vi "hammerbot blue.vi"   [LabVIEW 2010, in "HammerBot.lvrbt"]
uses:
  HammerBot.lvrbt
  <vilib>/NXT/Subs/MotorOutput.ctl
  <vilib>/NXT/Block Support/NXT_MessageMailbox.ctl
  <vilib>/NXT/Dual Mode Library/Motors/ResetMotor.vi
  <vilib>/NXT/Dual Mode Library/Motors/MotorOn.vi
  <vilib>/NXT/Dual Mode Library/Motors/Rotation.vi
  <vilib>/NXT/Dual Mode Library/Motors/MotorBrake.vi
  <vilib>/NXT/Dual Mode Library/Motors/MotorReverse.vi
types:
  T1 = typedef "MotorOutput.ctl" = u8
  T2 = typedef "NXT_MessageMailbox.ctl" = u8
  T3 = typedef "LVHSConnector.ctl" = cluster{"Hardware":string, "Flattened String":string}
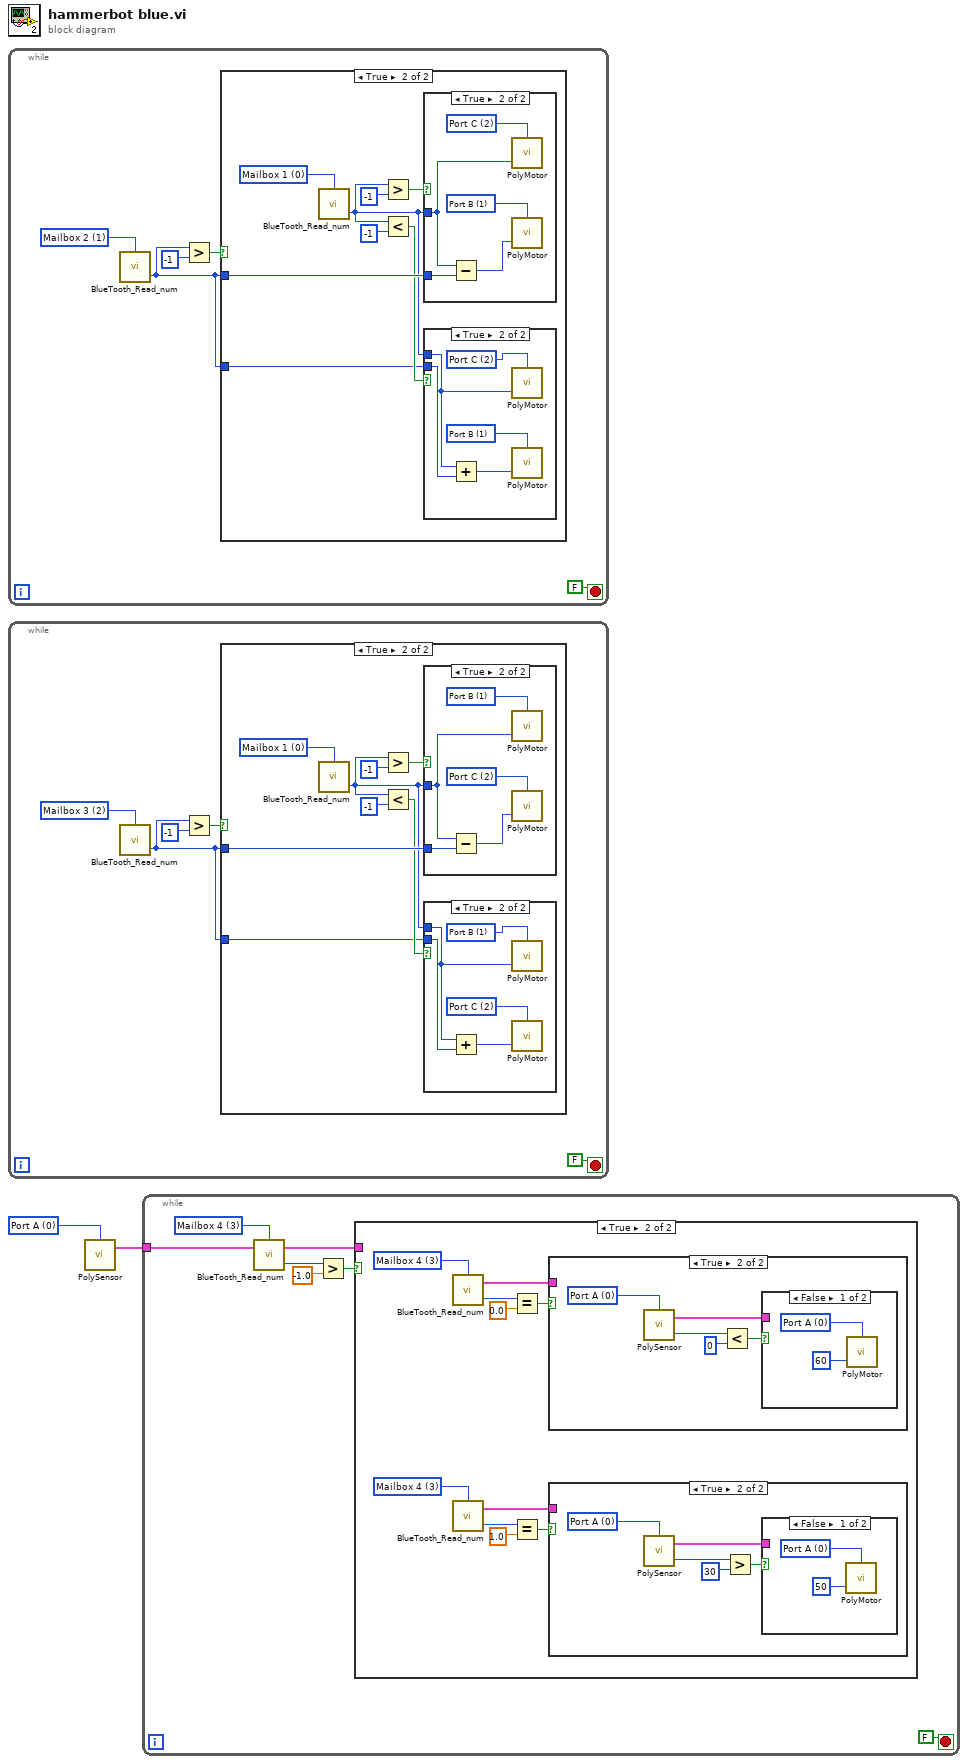
[diagram p0: block diagram]
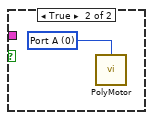
[diagram p10: hidden frame]
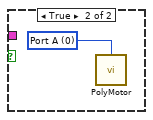
[diagram p12: hidden frame]
diagram:
  w1 = T1 0 items=["Port A"=0, "Port B"=1, "Port C"=2, "Ports A & B"=4, "Ports A & C"=5, "Ports B & C"=6, "All Ports"=3] ("Port (All Ports)")
  n1 = while {
    stop <- FALSE stop-if-true
    w7 = T2 1 items=["Mailbox 1", "Mailbox 2", "Mailbox 3", "Mailbox 4", "Mailbox 5", "Mailbox 6", "Mailbox 7", "Mailbox 8", "Mailbox 9", "Mailbox 10"] ("Mailbox")
    n2 = call <vilib>:"BlueTooth_Read_num.vi"("Mailbox"=w7) -> ("Message"=w3:i32)  [unwired: 2 in, 1 out]
    n3 = Greater?(x=w3, y=-1) -> (0:w5:bool)
    n4 = case shown="True" w5 {
      tunnel: w3 -> [_ w14]
      tunnel: w3 -> [_ w8]
      frame False {
      }
      frame True {
        w15 = T2 0 items=["Mailbox 1", "Mailbox 2", "Mailbox 3", "Mailbox 4", "Mailbox 5", "Mailbox 6", "Mailbox 7", "Mailbox 8", "Mailbox 9", "Mailbox 10"] ("Mailbox")
        n5 = call <vilib>:"BlueTooth_Read_num.vi"("Mailbox"=w15) -> ("Message"=w13:i32)  [unwired: 2 in, 1 out]
        n6 = Greater?(x=w13, y=-1) -> (0:w10:bool)
        n7 = Less?(x=w13, y=-1) -> (x < y?=w9:bool)
        n8 = case shown="True" w10 {
          tunnel: w13 -> [_ w24]
          tunnel: w14 -> [_ w21]
          frame False {
          }
          frame True {
            w25 = T1 1 items=["Port A"=0, "Port B"=1, "Port C"=2, "Ports A & B"=4, "Ports A & C"=5, "Ports B & C"=6, "All Ports"=3] ("Output Port (All Ports)")
            w22 = T1 2 items=["Port A"=0, "Port B"=1, "Port C"=2, "Ports A & B"=4, "Ports A & C"=5, "Ports B & C"=6, "All Ports"=3] ("Output Port (All Ports)")
            n9 = Subtract(x=w24, y=w21) -> (x-y=w23:i32)
            n10 = call-poly <vilib>:"PolyMotor.vi"("Power (75)"=w24, "Output Port (All Ports)"=w22) -> ()  [unwired: 2 in, 1 out]
            n11 = call-poly <vilib>:"PolyMotor.vi"("Power (75)"=w23, "Output Port (All Ports)"=w25) -> ()  [unwired: 2 in, 1 out]
          }
        }
        n12 = case shown="True" w9 {
          tunnel: w13 -> [_ w17]
          tunnel: w8 -> [_ w16]
          frame False {
          }
          frame True {
            w20 = T1 1 items=["Port A"=0, "Port B"=1, "Port C"=2, "Ports A & B"=4, "Ports A & C"=5, "Ports B & C"=6, "All Ports"=3] ("Output Port (All Ports)")
            w18 = T1 2 items=["Port A"=0, "Port B"=1, "Port C"=2, "Ports A & B"=4, "Ports A & C"=5, "Ports B & C"=6, "All Ports"=3] ("Output Port (All Ports)")
            n13 = Add(x=w17, y=w16) -> (x+y=w19:i32)
            n14 = call-poly <vilib>:"PolyMotor.vi"("Power (75)"=w17, "Output Port (All Ports)"=w18) -> ()  [unwired: 2 in, 1 out]
            n15 = call-poly <vilib>:"PolyMotor.vi"("Power (75)"=w19, "Output Port (All Ports)"=w20) -> ()  [unwired: 2 in, 1 out]
          }
        }
      }
    }
  }
  n16 = while {
    stop <- FALSE stop-if-true
    w30 = T2 2 items=["Mailbox 1", "Mailbox 2", "Mailbox 3", "Mailbox 4", "Mailbox 5", "Mailbox 6", "Mailbox 7", "Mailbox 8", "Mailbox 9", "Mailbox 10"] ("Mailbox")
    n17 = call <vilib>:"BlueTooth_Read_num.vi"("Mailbox"=w30) -> ("Message"=w26:i32)  [unwired: 2 in, 1 out]
    n18 = Greater?(x=w26, y=-1) -> (0:w28:bool)
    n19 = case shown="True" w28 {
      tunnel: w26 -> [_ w37]
      tunnel: w26 -> [_ w31]
      frame False {
      }
      frame True {
        w38 = T2 0 items=["Mailbox 1", "Mailbox 2", "Mailbox 3", "Mailbox 4", "Mailbox 5", "Mailbox 6", "Mailbox 7", "Mailbox 8", "Mailbox 9", "Mailbox 10"] ("Mailbox")
        n20 = call <vilib>:"BlueTooth_Read_num.vi"("Mailbox"=w38) -> ("Message"=w36:i32)  [unwired: 2 in, 1 out]
        n21 = Greater?(x=w36, y=-1) -> (0:w33:bool)
        n22 = Less?(x=w36, y=-1) -> (x < y?=w32:bool)
        n23 = case shown="True" w33 {
          tunnel: w36 -> [_ w47]
          tunnel: w37 -> [_ w44]
          frame False {
          }
          frame True {
            w48 = T1 2 items=["Port A"=0, "Port B"=1, "Port C"=2, "Ports A & B"=4, "Ports A & C"=5, "Ports B & C"=6, "All Ports"=3] ("Output Port (All Ports)")
            w45 = T1 1 items=["Port A"=0, "Port B"=1, "Port C"=2, "Ports A & B"=4, "Ports A & C"=5, "Ports B & C"=6, "All Ports"=3] ("Output Port (All Ports)")
            n24 = Subtract(x=w47, y=w44) -> (x-y=w46:i32)
            n25 = call-poly <vilib>:"PolyMotor.vi"("Power (75)"=w47, "Output Port (All Ports)"=w45) -> ()  [unwired: 2 in, 1 out]
            n26 = call-poly <vilib>:"PolyMotor.vi"("Power (75)"=w46, "Output Port (All Ports)"=w48) -> ()  [unwired: 2 in, 1 out]
          }
        }
        n27 = case shown="True" w32 {
          tunnel: w36 -> [_ w40]
          tunnel: w31 -> [_ w39]
          frame False {
          }
          frame True {
            w43 = T1 2 items=["Port A"=0, "Port B"=1, "Port C"=2, "Ports A & B"=4, "Ports A & C"=5, "Ports B & C"=6, "All Ports"=3] ("Output Port (All Ports)")
            w41 = T1 1 items=["Port A"=0, "Port B"=1, "Port C"=2, "Ports A & B"=4, "Ports A & C"=5, "Ports B & C"=6, "All Ports"=3] ("Output Port (All Ports)")
            n28 = Add(x=w40, y=w39) -> (x+y=w42:i32)
            n29 = call-poly <vilib>:"PolyMotor.vi"("Power (75)"=w40, "Output Port (All Ports)"=w41) -> ()  [unwired: 2 in, 1 out]
            n30 = call-poly <vilib>:"PolyMotor.vi"("Power (75)"=w42, "Output Port (All Ports)"=w43) -> ()  [unwired: 2 in, 1 out]
          }
        }
      }
    }
  }
  n31 = call-poly <vilib>:"PolySensor.vi"("Port (All Ports)"=w1) -> ("NXT"=w2:T3)  [unwired: 3 in]
  n32 = while {
    tunnel: w2 -> [w50]
    stop <- FALSE stop-if-true
    w54 = T2 3 items=["Mailbox 1", "Mailbox 2", "Mailbox 3", "Mailbox 4", "Mailbox 5", "Mailbox 6", "Mailbox 7", "Mailbox 8", "Mailbox 9", "Mailbox 10"] ("Mailbox")
    n33 = call <vilib>:"BlueTooth_Read_num.vi"("NXT"=w50, "Mailbox"=w54) -> ("Message"=w52:i32, "NXT"=w49:T3)  [unwired: 1 in]
    n34 = Greater?(x=w52, y=-1.0) -> (0:w51:bool)
    n35 = case shown="True" w51 {
      tunnel: w49 -> [_ _]
      frame False {
      }
      frame True {
        w60 = T2 3 items=["Mailbox 1", "Mailbox 2", "Mailbox 3", "Mailbox 4", "Mailbox 5", "Mailbox 6", "Mailbox 7", "Mailbox 8", "Mailbox 9", "Mailbox 10"] ("Mailbox")
        w65 = T2 3 items=["Mailbox 1", "Mailbox 2", "Mailbox 3", "Mailbox 4", "Mailbox 5", "Mailbox 6", "Mailbox 7", "Mailbox 8", "Mailbox 9", "Mailbox 10"] ("Mailbox")
        n36 = call <vilib>:"BlueTooth_Read_num.vi"("Mailbox"=w65) -> ("Message"=w62:i32, "NXT"=w61:T3)  [unwired: 2 in]
        n37 = call <vilib>:"BlueTooth_Read_num.vi"("Mailbox"=w60) -> ("Message"=w57:i32, "NXT"=w56:T3)  [unwired: 2 in]
        n38 = Equal?(x=w62, y=0.0) -> (x = y?=w63:bool)
        n39 = Equal?(x=w57, y=1.0) -> (x = y?=w58:bool)
        n40 = case shown="True" w63 {
          tunnel: w61 -> [_ _]
          frame False {
          }
          frame True {
            w75 = u8 0 items=["Port A", "Port B", "Port C"] ("Port (Port A)")
            n41 = call-poly <vilib>:"PolySensor.vi"("Port (Port A)"=w75) -> ("Angle of Rotation"=w78:i32, "NXT"=w74:T3)  [unwired: 2 in]
            n42 = Less?(x=w78, y=0) -> (x < y?=w76:bool)
            n43 = case shown="False" w76 {
              tunnel: w74 -> [_ _]
              frame False {
                w80 = T1 0 items=["Port A"=0, "Port B"=1, "Port C"=2, "Ports A & B"=4, "Ports A & C"=5, "Ports B & C"=6, "All Ports"=3] ("Output Port (All Ports)")
                n44 = call-poly <vilib>:"PolyMotor.vi"("Power (75)"=60, "Output Port (All Ports)"=w80) -> ()  [unwired: 2 in, 1 out]
              }
              frame True {
                w81 = T1 0 items=["Port A"=0, "Port B"=1, "Port C"=2, "Ports A & B"=4, "Ports A & C"=5, "Ports B & C"=6, "All Ports"=3] ("Output Port (All Ports)")
                n45 = call-poly <vilib>:"PolyMotor.vi"("Port (All Ports)"=w81) -> ()  [unwired: 3 in, 1 out]
              }
            }
          }
        }
        n46 = case shown="True" w58 {
          tunnel: w56 -> [_ _]
          frame False {
          }
          frame True {
            w68 = u8 0 items=["Port A", "Port B", "Port C"] ("Port (Port A)")
            n47 = call-poly <vilib>:"PolySensor.vi"("Port (Port A)"=w68) -> ("Angle of Rotation"=w70:i32, "NXT"=w66:T3)  [unwired: 2 in]
            n48 = Greater?(x=w70, y=30) -> (0:w69:bool)
            n49 = case shown="False" w69 {
              tunnel: w66 -> [_ _]
              frame False {
                w72 = T1 0 items=["Port A"=0, "Port B"=1, "Port C"=2, "Ports A & B"=4, "Ports A & C"=5, "Ports B & C"=6, "All Ports"=3] ("Output Port (All Ports)")
                n50 = call-poly <vilib>:"PolyMotor.vi"("Power (75)"=50, "Output Port (All Ports)"=w72) -> ()  [unwired: 2 in, 1 out]
              }
              frame True {
                w73 = T1 0 items=["Port A"=0, "Port B"=1, "Port C"=2, "Ports A & B"=4, "Ports A & C"=5, "Ports B & C"=6, "All Ports"=3] ("Output Port (All Ports)")
                n51 = call-poly <vilib>:"PolyMotor.vi"("Port (All Ports)"=w73) -> ()  [unwired: 3 in, 1 out]
              }
            }
          }
        }
      }
    }
  }
